vi "dust type.vi"(0 "Enable":bool=TRUE, 1 "Small?":bool, 2 "Sub vi?":bool, 5 "error in (no error)":errorcluster) -> (14 "Cancel 2":bool caption="Cancel", 15 "output cluster 2":T2 {"Batch" step=1; "Type" step=1; "Dust Source Builder:" items=["Keith Drake", "Nick Beaty", "Anthony Shu", "David James", "John Fontanese"]}, 16 "Dust Properties 2":T1, 18 "OK":bool, 19 "error out":errorcluster)   [LabVIEW 2013]
doc: "Displays a standard dialog box that prompts users to enter information, such as a user name and password.\n--------------------\n\nThis Express VI is configured as follows:\n\nMessage to Display to the User:Please Enter Experiment Settings Information For Database Storage.\nThe inputs are: \nNumber: Please Enter Group ID\nText Entry Box: Please Enter Tags:\nText Entry Box: Please Enter Experiment Description:"
uses:
  Controls/dust type.ctl
  Controls/source_builders.ctl
  Controls/dust_type_indicator.ctl
  <vilib>/Utility/miscctls.llb/LVPointTypeDef.ctl
  <vilib>/addons/database/Connection.llb/Conn Execute.vi
  <vilib>/addons/database/Recordset.llb/Rec Fetch Recordset Data (R).vi
  <vilib>/addons/database/Recordset.llb/Rec Destroy - Connection.vi
  <userlib>/_OpenG.lib/array/array.llb/Remove Duplicates from 1D Array (String)__ogtk.vi
  <userlib>/_OpenG.lib/array/array.llb/Search 1D Array (String)__ogtk.vi
  <userlib>/_OpenG.lib/array/array.llb/Index 1D Array Elements (I32)__ogtk.vi
  <userlib>/_OpenG.lib/array/array.llb/Conditional Auto-Indexing Tunnel (I32)__ogtk.vi
  <vilib>/addons/database/_DB Variant To Data/Database Variant To Data.xnode
  <vilib>/addons/database/NI_Database_API.lvlib
panel:
  in  "Transfer":bool caption="OK2"
  out "Comments":string[](array[string])
  out "Dust Properties":T1
  out "Dust Names":string[](array[string])
  out "Dust Weights":dbl[](array[numeric])
  out "Sizes":string[](array[string])
  out "Typical Weights":dbl[](array[numeric])
  out "Densities":dbl[](array[numeric])
  out "Batch Nos":i32[](array[numeric])
  out "Dust Types":i32[](array[numeric])
  out "Dust Type Ids":i32[](array[numeric])
  in  "Controls":T2 {"Batch" min=1 max=2 step=1; "Type" min=1 max=10 step=1; "Dust Source Builder:" items=["Keith Drake", "Nick Beaty", "Anthony Shu", "David James", "John Fontanese"]}
  in  "Create New":bool caption="OK2"
  in  "Cancel":bool
  in  "Update":bool caption="OK1"
  # "Please Enter Dust Information For Storage in the CCLDAS Database."
  # "Dust Information"
  # "Dust Information"
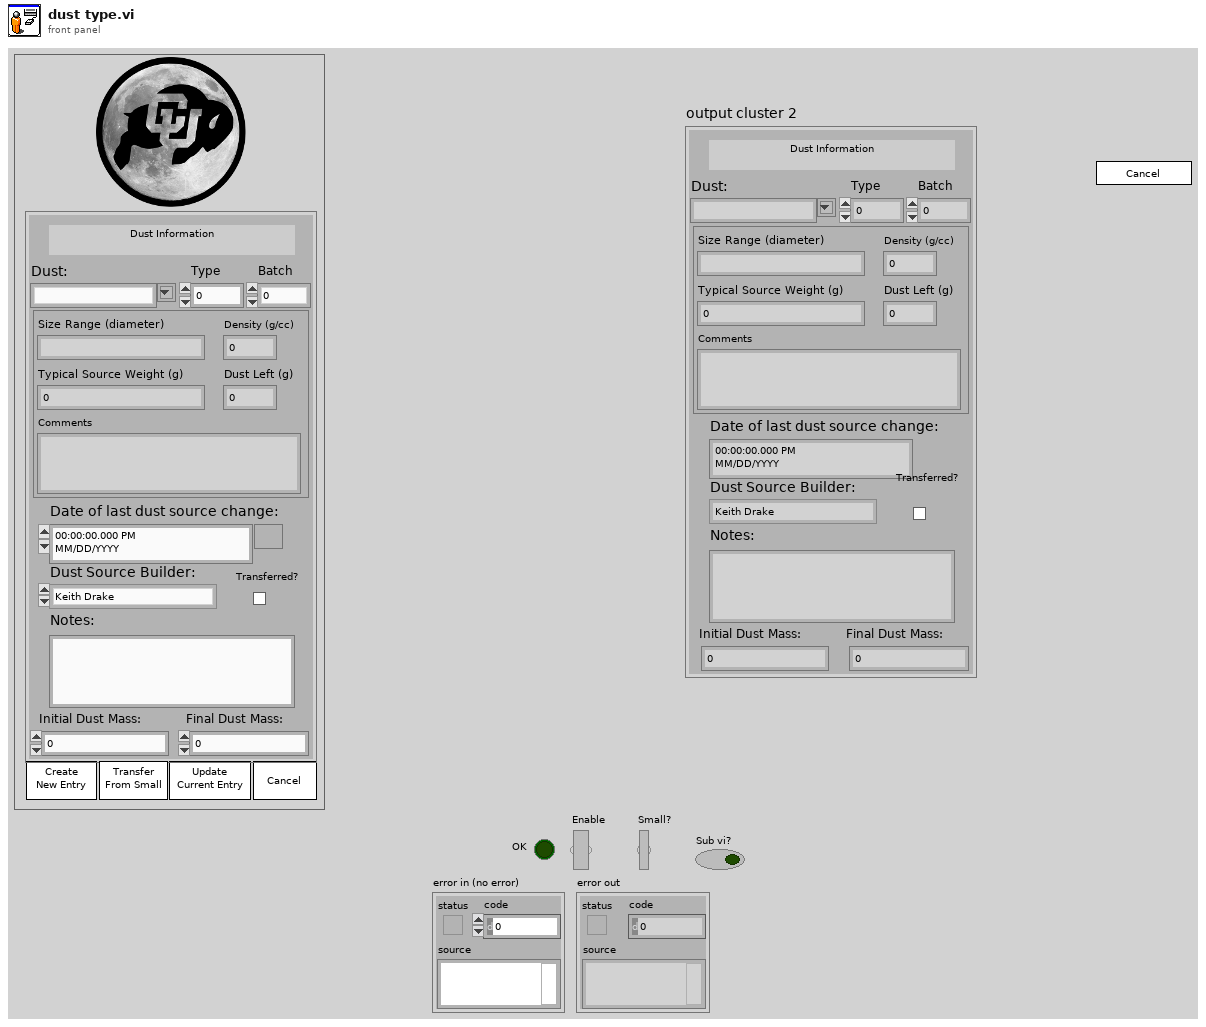
[diagram p1: front panel]
types:
  T1 = typedef "dust_type_indicator.ctl" = cluster{"Size Range (diameter)":string, "Density (g/cc)":dbl, "Typical Source Weight (g)":dbl, "Dust Left (g)":dbl, "Comments":string}
  T2 = typedef "dust type.ctl" = cluster{"Dust info id":u16, "Integer Timestamp":i64, "Dust:":string, "Dust Source Builder:":T3, "Notes:":string, "Date of last dust source change:":timestamp, "Initial Dust Mass:":dbl, "Final Dust Mass:":dbl, "Type":u16, "Batch":u16, "dust type id":u16, "Transferred?":bool}
  T3 = typedef "source_builders.ctl" = u16
  T4 = typedef "LVPointTypeDef.ctl" = cluster{"Horizontal":i16, "Vertical":i16}
  T5 = enum8{"Enabled", "Disabled", "Disabled and Grayed Out"}
  T6 = enum32{"Invalid", "Standard", "Closed", "Hidden", "Minimized", "Maximized"}
  T7 = cluster{"Dust info id":u16, "Integer Timestamp":i64, "dust type id":u16, "Dust Source Builder:":u16, "Notes:":string, "Initial Dust Mass:":dbl, "Final Dust Mass:":dbl, "shot count":u16, "run time":dbl, "From Small\nAccelerator":bool}
  T8 = typedef "NI_Database_API.lvlib/Conn ObjectReference.ctl" = refnum<k1>
  T9 = typedef "NI_Database_API.lvlib/Rec ObjectReference.ctl" = refnum<k1>
  T10 = cluster{"Dust event id":dbl, "Integer Time":i64, "dust type id":u16, "Dust Source Builder:":T3, "Notes:":string, "Initial Dust Mass:":dbl, "Dust event id":dbl, i16}
  T11 = cluster{"Dust event id":dbl, "Integer Time":i64, "dust type id":u16, "Dust Source Builder:":u16, "Notes:":string, "Initial Dust Mass:":dbl, "Final Dust Mass:":dbl, "shot count":u16, "run time":dbl, i16}
  T12 = cluster{"data":string, "data":dbl, "data":dbl, "data":dbl, "data":string}
  T13 = cluster{"Dust info id":u16, "Integer Timestamp":i64, "dust type id":u16, "Dust Source Builder:":T3, "Notes:":string, "Initial Dust Mass:":dbl, "Final Dust Mass:":dbl, i16}
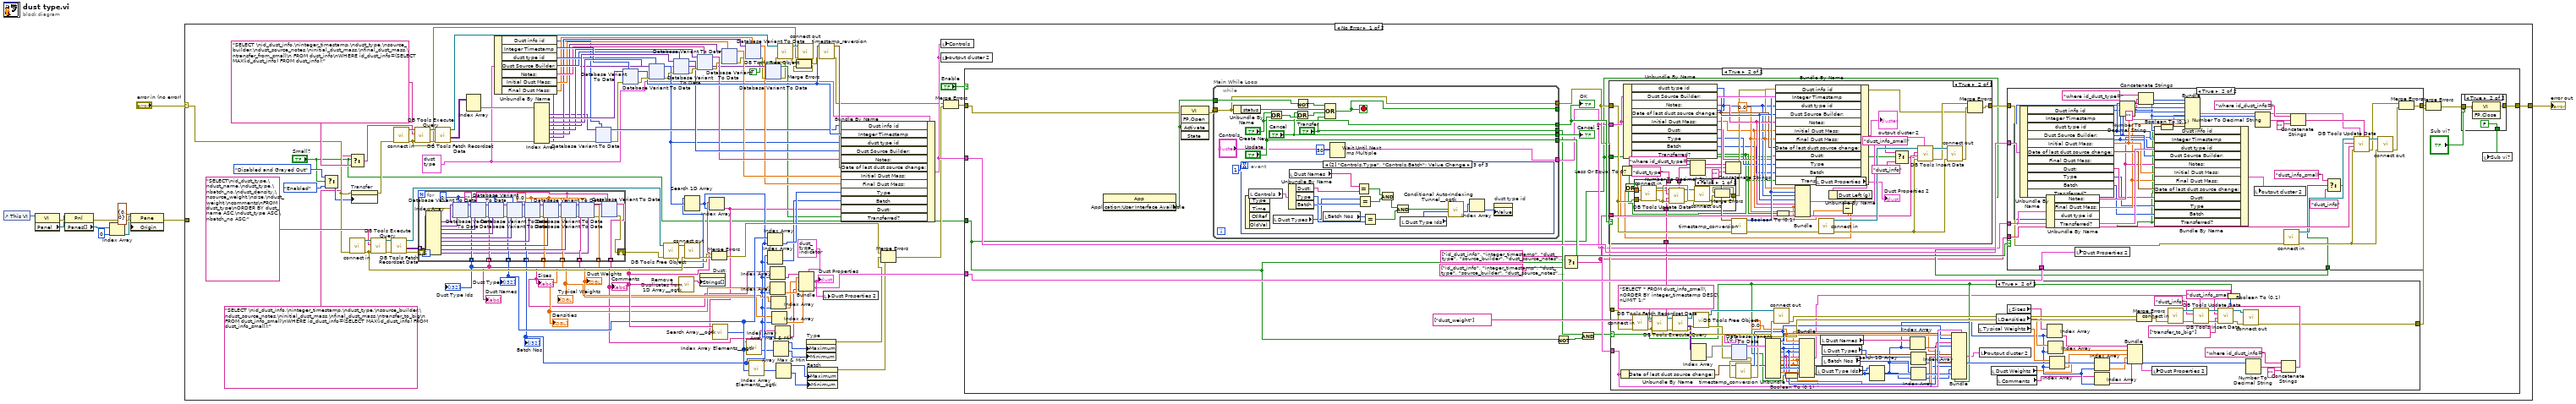
[diagram p0: block diagram]
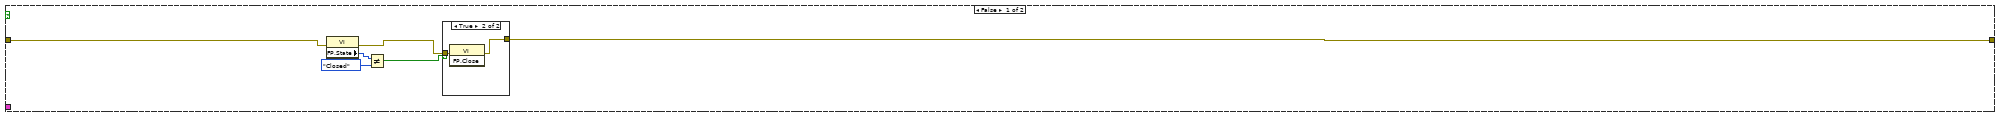
[diagram p2: hidden frame]
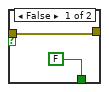
[diagram p4: hidden frame]
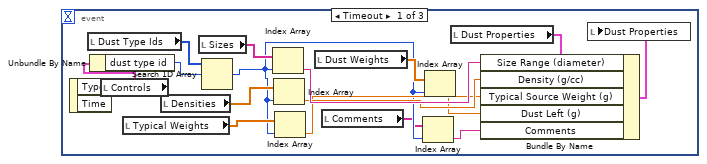
[diagram p7: hidden frame]
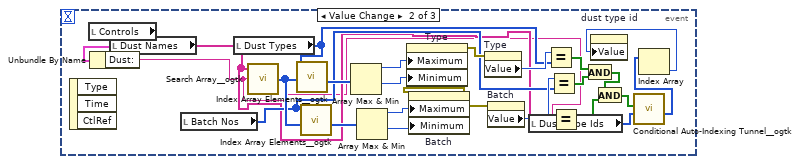
[diagram p8: hidden frame]
diagram:
  n1 = control-ref of="This VI"() -> (w9:refnum<vi>)
  n2 = property class="VI"(reference=w9) -> (error out=w8:errorcluster, "Panel"=w7:refnum<vi>)  [unwired: 1 in, 1 out]
  n3 = property class="Pnl"(reference=w7, error in=w8) -> (error out=w6:errorcluster, "Panes[]"=w5:refnum<vi>[])  [unwired: 1 out]
  n4 = Index Array(array=w5, index=0) -> (element=w3:refnum<vi>)
  n5 = property class="Pane"(reference=w3, error in=w6, "Origin"=T4 {"Horizontal"=0, "Vertical"=0}) -> (error out=w1:errorcluster)  [unwired: 1 out]
  n6 = case shown="No Error" "error in (no error)" {
    selector: "error in (no error)" -> [w25 w1275]
    tunnel: [w110 w1275] -> w10
    tunnel: w1 -> [_ _]
    frame No Error {
      w32 = T2 {"Dust info id"=0, "Integer Timestamp"=0, "Dust:"="", "Dust Source Builder:"=0, "Notes:"="", "Date of last dust source change:"=timestamp(0 s since 1904-01-01), "Initial Dust Mass:"=0.0, "Final Dust Mass:"=0.0, "Type"=0, "Batch"=0, "dust type id"=0, "Transferred?"=FALSE} ("Controls")
      n7 = Select(t=T5."Disabled and Grayed Out" ("Disabled"), s="Small?", f=T5."Enabled" ("Disabled")) -> (s? t:f=w21:T5)
      n8 = Select(t="SELECT \nid_dust_info,\ninteger_timestamp,\ndust_type,\nsource_builder,\ndust_source_notes,\ninitial_dust_mass,\nfinal_dust_mass,\ntransfer_to_big\n FROM dust_info_small\nWHERE id_dust_info=(SELECT MAX(id_dust_info) FROM dust_info_small);" ("SQL query"), s="Small?", f="SELECT \nid_dust_info,\ninteger_timestamp,\ndust_type,\nsource_builder,\ndust_source_notes,\ninitial_dust_mass,\nfinal_dust_mass,\ntransfer_from_small\n FROM dust_info\nWHERE id_dust_info=(SELECT MAX(id_dust_info) FROM dust_info);" ("SQL query")) -> (s? t:f=w26:string)
      n9 = call "connect in.vi"("error in (no error)"=w25) -> ("error out"=w69:errorcluster, "Database Connection"=w76:T8)  [unwired: 6 in, 1 out]
      n10 = property on="Transfer" class="Bool (strict)"(error in=w25, "DisabledEnum"=w21) -> (error out=w24:errorcluster)  [unwired: 1 in, 1 out]
      n11 = call-poly <vilib>:"DB Tools Execute Query.vi"("error in (no error)"=w69, "SQL query"="SELECT\nid_dust_type,\ndust_name,\ndust_type,\nbatch_no,\ndust_density,\nsource_weight,\nsize,\ndust_weight,\ncomments\nFROM dust_type\nORDER BY dust_name ASC,\ndust_type ASC,\nbatch_no ASC;", "connection reference"=w76) -> ("error out"=w78:errorcluster, "recordset reference"=w77:T9)  [unwired: 5 in]
      n12 = call-poly <vilib>:"DB Tools Fetch Recordset Data.vi"("error in (no error)"=w78, "recordset reference"=w77) -> ("error out"=w73:errorcluster, "recordset data"=w74:variant[][], "recordset reference out"=w70:T9)  [unwired: 3 in]
      n13 = call "connect in.vi"("error in (no error)"=w24) -> ("error out"=w68:errorcluster, "Database Connection"=w111:T8)  [unwired: 6 in, 1 out]
      n14 = call-poly <vilib>:"DB Tools Execute Query.vi"("error in (no error)"=w68, "SQL query"=w26, "connection reference"=w111) -> ("error out"=w113:errorcluster, "recordset reference"=w112:T9)  [unwired: 5 in]
      n15 = for {
        tunnel: w74 -> [w179] mode=indexing
        shift-right: [w149] -> w71
        shift-left: w73 -> [w170]
        tunnel: [w160] -> w61 mode=indexing
        tunnel: [w159] -> w59 mode=indexing
        tunnel: [w158] -> w57 mode=indexing
        tunnel: [w157] -> w56 mode=indexing
        tunnel: [w156] -> w53 mode=indexing
        tunnel: [w155] -> w54 mode=indexing
        tunnel: [w154] -> w52 mode=indexing
        tunnel: [w153] -> w55 mode=indexing
        tunnel: [w148] -> w34 mode=indexing
        w161 = 0.0
        w152 = ""
        w162 = 0
        n16 = Index Array(array=w179) -> (element #1=w178:variant, element #2=w177:variant, element #3=w176:variant, element #4=w175:variant, element #5=w174:variant, element #6=w173:variant, element #7=w172:variant, element #8=w171:variant, element #9=w151:variant)  [unwired: 9 in]
        n17 = xnode "Database Variant To Data"("database variant"=w178, "error in (no error)"=w170, "type"=w162) -> ("data"=w160:i32, "error out"=w169:errorcluster)
        n18 = xnode "Database Variant To Data"("database variant"=w177, "error in (no error)"=w169, "type"=w152) -> ("data"=w159:string, "error out"=w168:errorcluster)
        n19 = xnode "Database Variant To Data"("database variant"=w176, "error in (no error)"=w168, "type"=w162) -> ("data"=w158:i32, "error out"=w167:errorcluster)
        n20 = xnode "Database Variant To Data"("database variant"=w175, "error in (no error)"=w167, "type"=w162) -> ("data"=w157:i32, "error out"=w166:errorcluster)
        n21 = xnode "Database Variant To Data"("database variant"=w174, "error in (no error)"=w166, "type"=w161) -> ("data"=w156:dbl, "error out"=w165:errorcluster)
        n22 = xnode "Database Variant To Data"("database variant"=w173, "error in (no error)"=w165, "type"=w161) -> ("data"=w155:dbl, "error out"=w164:errorcluster)
        n23 = xnode "Database Variant To Data"("database variant"=w172, "error in (no error)"=w164, "type"=w152) -> ("data"=w154:string, "error out"=w163:errorcluster)
        n24 = xnode "Database Variant To Data"("database variant"=w171, "error in (no error)"=w163, "type"=w161) -> ("data"=w153:dbl, "error out"=w150:errorcluster)
        n25 = xnode "Database Variant To Data"("database variant"=w151, "error in (no error)"=w150, "type"=w152) -> ("data"=w148:string, "error out"=w149:errorcluster)
      }
      "Dust Type Ids" <- w61
      "Dust Types" <- w57
      "Batch Nos" <- w56
      "Densities" <- w53
      "Typical Weights" <- w54
      "Sizes" <- w52
      "Dust Weights" <- w55
      "Dust Names" <- w59
      "Comments" <- w34
      n26 = call-poly <vilib>:"DB Tools Fetch Recordset Data.vi"("error in (no error)"=w113, "recordset reference"=w112) -> ("error out"=w80:errorcluster, "recordset data"=w98:variant[][], "recordset reference out"=w114:T9)  [unwired: 3 in]
      n27 = Index Array(array=w98) -> (element=w97:variant[])  [unwired: 2 in]
      n28 = Unbundle By Name(w32) -> ("Dust info id"=w17:u16, "Integer Timestamp"=w104:i64, "dust type id"=w103:u16, "Dust Source Builder:"=w102:T3, "Notes:"=w100:string, "Initial Dust Mass:"=w89:dbl, "Final Dust Mass:"=w87:dbl)
      n29 = Index Array(array=w97) -> (element #1=w82:variant, element #2=w109:variant, element #3=w108:variant, element #4=w106:variant, element #5=w101:variant, element #6=w90:variant, element #7=w85:variant, element #8=w19:variant)  [unwired: 8 in]
      n30 = xnode "Database Variant To Data"("database variant"=w82, "error in (no error)"=w80, "type"=w17) -> ("data"=w81:u16, "error out"=w79:errorcluster)
      n31 = xnode "Database Variant To Data"("database variant"=w109, "error in (no error)"=w79, "type"=w104) -> ("data"=w95:i64, "error out"=w107:errorcluster)
      n32 = xnode "Database Variant To Data"("database variant"=w108, "error in (no error)"=w107, "type"=w103) -> ("data"=w62:u16, "error out"=w105:errorcluster)
      n33 = call-poly <vilib>:"DB Tools Free Object.vi"("error in (no error)"=w71, "recordset reference"=w70) -> ("error out"=w63:errorcluster, "connection reference"=w72:T8)  [unwired: 8 in]
      n34 = xnode "Database Variant To Data"("database variant"=w106, "error in (no error)"=w105, "type"=w102) -> ("data"=w92:T3, "error out"=w99:errorcluster)
      n35 = call-poly <userlib>:"Remove Duplicates from 1D Array__ogtk.vi"("Input Array"=w59) -> ("Output Array"=w60:string[])  [unwired: 1 out]
      n36 = call "connect out.vi"("error in (no error)"=w69, "connection reference"=w72) -> ("error out"=w64:errorcluster)  [unwired: 9 in]
      n37 = Search 1D Array(1D array=w61, element=w62) -> (index of element=w35:i32)  [unwired: 1 in]
      n38 = xnode "Database Variant To Data"("database variant"=w101, "error in (no error)"=w99, "type"=w100) -> ("data"=w91:string, "error out"=w84:errorcluster)
      n39 = property on="Dust:" class="CmbBox"("Strings[]"=w60) -> ()  [unwired: 2 in, 2 out]
      n40 = Index Array(array=w59, index=w35) -> (element=w28:string)
      n41 = Merge Errors(w63, w64) -> (w41:errorcluster)
      n42 = call-poly <userlib>:"Search Array__ogtk.vi"("Array"=w59, "Element Data"=w28) -> ("Indices of Elements"=w58:i32[])  [unwired: 7 in]
      n43 = xnode "Database Variant To Data"("database variant"=w90, "error in (no error)"=w84, "type"=w89) -> ("data"=w88:dbl, "error out"=w83:errorcluster)
      n44 = xnode "Database Variant To Data"("database variant"=w85, "error in (no error)"=w83, "type"=w87) -> ("data"=w86:dbl, "error out"=w14:errorcluster)
      n45 = call-poly <userlib>:"Index Array Elements__ogtk.vi"("indices"=w58, "array"=w57) -> ("elements"=w47:i32[])  [unwired: 9 in]
      n46 = call-poly <userlib>:"Index Array Elements__ogtk.vi"("indices"=w58, "array"=w56) -> ("elements"=w46:i32[])  [unwired: 9 in]
      n47 = xnode "Database Variant To Data"("database variant"=w19, "error in (no error)"=w14, "type"=TRUE ("Small?")) -> ("data"=w15:bool, "error out"=w13:errorcluster)
      n48 = Index Array(array=w56, index=w35) -> (element=w36:i32)
      n49 = Index Array(array=w57, index=w35) -> (element=w37:i32)
      n50 = Index Array(array=w52, index=w35) -> (element=w51:string)
      n51 = Index Array(array=w53, index=w35) -> (element=w50:dbl)
      n52 = Index Array(array=w54, index=w35) -> (element=w49:dbl)
      n53 = Index Array(array=w55, index=w35) -> (element=w48:dbl)
      n54 = Array Max & Min(array=w47) -> (max value=w45:i32, min value=w44:i32)  [unwired: 2 out]
      n55 = Index Array(array=w34, index=w35) -> (element=w33:string)
      n56 = Array Max & Min(array=w46) -> (max value=w43:i32, min value=w42:i32)  [unwired: 2 out]
      n57 = call-poly <vilib>:"DB Tools Free Object.vi"("error in (no error)"=w13, "recordset reference"=w114) -> ("error out"=w67:errorcluster, "connection reference"=w115:T8)  [unwired: 8 in]
      n58 = call "connect out.vi"("error in (no error)"=w68, "connection reference"=w115) -> ("error out"=w65:errorcluster)  [unwired: 9 in]
      n59 = Merge Errors(w67, w65) -> (w66:errorcluster)
      n60 = Bundle(cluster=T1 {"Size Range (diameter)"="60 nm - 10 µm", "Density (g/cc)"=7874.0, "Typical Source Weight (g)"=1.2000000476837158, "Dust Left (g)"=0.9300000071525574, "Comments"="8:1 mix of Iron-8-1 and Iron-4-1."} ("Dust Properties"), "Size Range (diameter)"=w51, "Density (g/cc)"=w50, "Typical Source Weight (g)"=w49, "Dust Left (g)"=w48, "Comments"=w33) -> (w31:T1)
      "Dust Properties" <- w31
      n61 = property on="Type" class="DigNum (strict)"("Maximum"=w45, "Minimum"=w44) -> (error out=w30:errorcluster)  [unwired: 2 in, 1 out]
      n62 = property on="Batch" class="DigNum (strict)"("Maximum"=w43, "Minimum"=w42) -> (error out=w29:errorcluster)  [unwired: 2 in, 1 out]
      n63 = call "timestamp_reversion.vi"("error in (no error)"=w66, "Integer Timestamp"=w95) -> ("error out"=w39:errorcluster, "time stamp"=w93:timestamp)  [unwired: 7 in]
      n64 = local write "Dust Properties 2"(w31) -> ()
      n65 = Bundle By Name(cluster=w32, "Dust info id"=w81, "Integer Timestamp"=w95, "dust type id"=w62, "Dust Source Builder:"=w92, "Notes:"=w91, "Date of last dust source change:"=w93, "Initial Dust Mass:"=w88, "Final Dust Mass:"=w86, "Type"=w37, "Batch"=w36, "Dust:"=w28, "Transferred?"=w15) -> (w94:T2)
      n66 = Merge Errors(w41, w30, w29) -> (w38:errorcluster)
      n67 = local write "Controls"(w94) -> ()
      n68 = local write "output cluster 2"(w94) -> ()
      n69 = Merge Errors(w39, w38) -> (w40:errorcluster)
      n70 = case shown="True" "Enable" {
        tunnel: w40 -> [w568 w582]
        tunnel: [w569 w596] -> w110
        tunnel: w94 -> [_ w592]
        tunnel: w31 -> [_ w589]
        tunnel: "Small?" -> [_ w578]
        frame False {
          n71 = property class="VI"(error in=w568) -> (error out=w567:errorcluster, "FP.State"=w566:T6)  [unwired: 1 in, 1 out]
          n72 = Not Equal?(x=w566, y=T6."Closed") -> (x != y?=w564:bool)
          n73 = case shown="True" w564 {
            tunnel: [w570 w572] -> w569
            tunnel: w567 -> [w570 w571]
            frame False {
            }
            frame True {
              n74 = invoke class="VI" method="FP.Close"(error in=w571) -> (error out=w572:errorcluster)  [unwired: 2 in, 2 out]
            }
          }
        }
        frame True {
          n75 = property class="App"() -> ("Application:User Interface Available"=w591:bool)  [unwired: 2 in, 2 out]
          n76 = invoke class="VI" method="FP.Open"(error in=w582, "Activate"=w591) -> (error out=w597:errorcluster)  [unwired: 3 in, 4 out]
          n77 = while "Main While Loop" {
            tunnel: w591 -> [w1036]
            tunnel: [w1032] -> _
            tunnel: w597 -> [w1030]
            tunnel: [w1030] -> w587
            tunnel: ["Cancel"] -> w595
            tunnel: ["Controls"] -> w586
            tunnel: ["Update"] -> w594
            tunnel: ["Create New"] -> w588
            tunnel: ["Transfer"] -> w579
            stop <- w1032 stop-if-true
            n78 = Unbundle By Name(w1030) -> ("status"=w1033:bool)
            n79 = event shown="[2] \"Controls.Type\", \"Controls.Batch\": Value Change" {
              selector: _ -> [_ _ _]
              dyn-events: _ -> [_ _ _]
              timeout: 1 -> [_ _ _]
              event Timeout {
                n80 = event-data() -> ()  [unwired: 1 in, 2 out]
                n81 = local read "Dust Type Ids"() -> (w1053:i32[])
                n82 = local read "Controls"() -> (w1039:T2)
                n83 = Unbundle By Name(w1039) -> ("dust type id"=w1054:u16)
                n84 = local read "Typical Weights"() -> (w1050:dbl[])
                n85 = local read "Densities"() -> (w1051:dbl[])
                n86 = local read "Sizes"() -> (w1052:string[])
                n87 = Search 1D Array(1D array=w1053, element=w1054) -> (index of element=w1042:i32)  [unwired: 1 in]
                n88 = Index Array(array=w1052, index=w1042) -> (element=w1046:string)
                n89 = Index Array(array=w1051, index=w1042) -> (element=w1045:dbl)
                n90 = Index Array(array=w1050, index=w1042) -> (element=w1044:dbl)
                n91 = local read "Dust Weights"() -> (w1049:dbl[])
                n92 = local read "Comments"() -> (w1041:string[])
                n93 = Index Array(array=w1041, index=w1042) -> (element=w1040:string)
                n94 = Index Array(array=w1049, index=w1042) -> (element=w1043:dbl)
                n95 = local read "Dust Properties"() -> (w1047:T1)
                n96 = Bundle By Name(cluster=w1047, "Size Range (diameter)"=w1046, "Density (g/cc)"=w1045, "Typical Source Weight (g)"=w1044, "Dust Left (g)"=w1043, "Comments"=w1040) -> (w1048:T1)
                n97 = local write "Dust Properties"(w1048) -> ()
              }
              event Value Change {
                n98 = event-data() -> ()  [unwired: 1 in, 3 out]
                n99 = local read "Controls"() -> (w1056:T2)
                n100 = Unbundle By Name(w1056) -> ("Dust:"=w1055:string)
                n101 = local read "Dust Names"() -> (w1065:string[])
                n102 = local read "Batch Nos"() -> (w1066:i32[])
                n103 = local read "Dust Types"() -> (w1068:i32[])
                n104 = call-poly <userlib>:"Search Array__ogtk.vi"("Array"=w1065, "Element Data"=w1055) -> ("Indices of Elements"=w1077:i32[])  [unwired: 7 in]
                n105 = call-poly <userlib>:"Index Array Elements__ogtk.vi"("indices"=w1077, "array"=w1068) -> ("elements"=w1076:i32[])  [unwired: 9 in]
                n106 = call-poly <userlib>:"Index Array Elements__ogtk.vi"("indices"=w1077, "array"=w1066) -> ("elements"=w1078:i32[])  [unwired: 9 in]
                n107 = Array Max & Min(array=w1076) -> (max value=w1075:i32, min value=w1074:i32)  [unwired: 2 out]
                n108 = Array Max & Min(array=w1078) -> (max value=w1073:i32, min value=w1072:i32)  [unwired: 2 out]
                n109 = property on="Type" class="DigNum (strict)"("Maximum"=w1075, "Minimum"=w1074) -> (error out=w1071:errorcluster)  [unwired: 2 in, 1 out]
                n110 = property on="Batch" class="DigNum (strict)"("Maximum"=w1073, "Minimum"=w1072) -> (error out=w1070:errorcluster)  [unwired: 2 in, 1 out]
                n111 = property on="Type" class="DigNum (strict)"(error in=w1071) -> ("Value"=w1069:u16)  [unwired: 1 in, 2 out]
                n112 = property on="Batch" class="DigNum (strict)"(error in=w1070) -> ("Value"=w1067:u16)  [unwired: 1 in, 2 out]
                n113 = local read "Dust Type Ids"() -> (w1059:i32[])
                n114 = Equal?(x=w1069, y=w1068) -> (x = y?=w1064:bool[])
                n115 = Equal?(x=w1067, y=w1066) -> (x = y?=w1063:bool[])
                n116 = Equal?(x=w1055, y=w1065) -> (x = y?=w1061:bool[])
                n117 = And(x=w1064, y=w1063) -> (x .and. y?=w1062:bool[])
                n118 = And(x=w1062, y=w1061) -> (x .and. y?=w1060:bool[])
                n119 = call-poly <userlib>:"Conditional Auto-Indexing Tunnel__ogtk.vi"("Array in"=w1059, "Elements to keep"=w1060) -> ("Filtered Array out"=w1058:i32[])  [unwired: 5 in]
                n120 = Index Array(array=w1058) -> (element=w1057:i32)  [unwired: 1 in]
                n121 = property on="dust type id" class="Ring (strict)"("Value"=w1057) -> ()  [unwired: 2 in, 2 out]
              }
              event Value Change {
                n122 = event-data() -> ()  [unwired: 1 in, 4 out]
                n123 = local read "Controls"() -> (w1080:T2)
                n124 = local read "Dust Types"() -> (w1089:i32[])
                n125 = Unbundle By Name(w1080) -> ("Dust:"=w1079:string, "Type"=w1093:u16, "Batch"=w1092:u16)
                n126 = local read "Dust Names"() -> (w1091:string[])
                n127 = local read "Batch Nos"() -> (w1090:i32[])
                n128 = Equal?(x=w1091, y=w1079) -> (x = y?=w1088:bool[])
                n129 = Equal?(x=w1089, y=w1093) -> (x = y?=w1087:bool[])
                n130 = Equal?(x=w1090, y=w1092) -> (x = y?=w1085:bool[])
                n131 = And(x=w1088, y=w1087) -> (x .and. y?=w1086:bool[])
                n132 = And(x=w1086, y=w1085) -> (x .and. y?=w1084:bool[])
                n133 = local read "Dust Type Ids"() -> (w1083:i32[])
                n134 = call-poly <userlib>:"Conditional Auto-Indexing Tunnel__ogtk.vi"("Array in"=w1083, "Elements to keep"=w1084) -> ("Filtered Array out"=w1082:i32[])  [unwired: 5 in]
                n135 = Index Array(array=w1082) -> (element=w1081:i32)  [unwired: 1 in]
                n136 = property on="dust type id" class="Ring (strict)"("Value"=w1081) -> ()  [unwired: 2 in, 2 out]
              }
            }
            n137 = Or(x="Create New", y="Update") -> (x .or. y?=w1037:bool)
            n138 = Or(x="Cancel", y=w1037) -> (x .or. y?=w1034:bool)
            n139 = Not(x=w1036) -> (.not. x?=w1035:bool)
            n140 = Compound Arithmetic op=OR(w1035, w1033, w1034, "Transfer") -> (w1032:bool)
            n141 = Wait Until Next ms Multiple(millisecond multiple=u32 50) -> ()  [unwired: 1 out]
          }
          "OK" <- w588
          "Cancel 2" <- w595
          n142 = Not(x=w578) -> (.not. x?=w580:bool)
          n143 = Select(t=string[] ["id_dust_info", "integer_timestamp", "dust_type", "source_builder", "dust_source_notes", "initial_dust_mass", "final_dust_mass", "transfer_to_big"] ("columns"), s=w578, f=string[] ["id_dust_info", "integer_timestamp", "dust_type", "source_builder", "dust_source_notes", "initial_dust_mass", "final_dust_mass", "transfer_from_small"] ("columns")) -> (s? t:f=w575:string[])
          n144 = And(x=w579, y=w580) -> (x .and. y?=w581:bool)
          n145 = case shown="True" w588 {
            tunnel: w587 -> [w1094 w1118]
            tunnel: [w1094 w1122] -> w593
            tunnel: w586 -> [_ w1128]
            tunnel: w575 -> [_ w1121]
            tunnel: string[] ["dust_weight"] -> [_ w1116]
            tunnel: w578 -> [_ w1097]
            frame False {
            }
            frame True {
              w1119 = 0.0 ("Dust event id")
              n146 = Unbundle By Name(w1128) -> ("dust type id"=w1105:u16, "Dust Source Builder:"=w1125:T3, "Notes:"=w1124:string, "Date of last dust source change:"=w1120:timestamp, "Initial Dust Mass:"=w1113:dbl, "Dust:"=w1104:string, "Type"=w1103:u16, "Batch"=w1102:u16, "Transferred?"=w1100:bool)
              n147 = Number To Decimal String(number=w1105) -> (decimal integer string=w1108:string)  [unwired: 1 in]
              n148 = Concatenate Strings("where id_dust_type=" ("condition"), w1108, "" ("string")) -> (w1106:string)
              n149 = call "timestamp_conversion.vi"("error in (no error)"=w1118, "Time Stamp"=w1120) -> ("error out"=w1134:errorcluster, "Integer Time"=w1126:i64)  [unwired: 7 in]
              n150 = Bundle By Name(cluster=w1128, "Dust info id"=w1119, "Integer Timestamp"=w1126, "dust type id"=w1105, "Dust Source Builder:"=w1125, "Notes:"=w1124, "Initial Dust Mass:"=w1113, "Final Dust Mass:"=w1119, "Date of last dust source change:"=w1120, "Dust:"=w1104, "Type"=w1103, "Batch"=w1102, "Transferred?"=w1100) -> (→"output cluster 2":T2)
              n151 = Boolean To (0,1)(Boolean=w1100) -> (0, 1=w1095:i16)
              n152 = Bundle("Dust event id"=w1119, "Integer Time"=w1126, "dust type id"=w1105, "Dust Source Builder:"=w1125, "Notes:"=w1124, "Initial Dust Mass:"=w1113, "Dust event id"=w1119, w1095) -> (w1123:T10)  [unwired: 1 in]
              n153 = local read "Dust Properties"() -> (w1114:T1)
              "Dust Properties 2" <- w1114
              n154 = call "connect in.vi"("error in (no error)"=w1134) -> ("error out"=w1131:errorcluster, "Database Connection"=w1133:T8)  [unwired: 6 in, 1 out]
              n155 = Unbundle By Name(w1114) -> ("Dust Left (g)"=w1110:dbl)
              n156 = Less Or Equal To 0?(x=w1110) -> (x <= 0?=w1111:bool)
              n157 = Or(x=w1111, y=w1100) -> (x .or. y?=w1101:bool)
              n158 = Subtract(x=w1110, y=w1113) -> (x-y=w1112:dbl)
              n159 = case shown="False" w1101 {
                tunnel: [w1142 w1146] -> w1117
                tunnel: w1118 -> [w1141 w1146]
                tunnel: w1116 -> [w1140 _]
                tunnel: "dust_type" -> [w1139 _]
                tunnel: w1112 -> [w1136 _]
                tunnel: w1106 -> [w1135 _]
                frame False {
                  n160 = call "connect in.vi"("error in (no error)"=w1141) -> ("error out"=w1145:errorcluster, "Database Connection"=w1138:T8)  [unwired: 6 in, 1 out]
                  n161 = call <vilib>:"DB Tools Update Data.vi"("condition"=w1135, "data"=w1136, "error in (no error)"=w1145, "columns"=w1140, "table"=w1139, "connection reference"=w1138) -> ("error out"=w1144:errorcluster, "connection reference out"=w1137:T8)  [unwired: 4 in]
                  n162 = call "connect out.vi"("error in (no error)"=w1145, "connection reference"=w1137) -> ("error out"=w1143:errorcluster)  [unwired: 9 in]
                  n163 = Merge Errors(w1143, w1144) -> (w1142:errorcluster)
                }
                frame True {
                }
              }
              n164 = Select(t="dust_info_small" ("table"), s=w1097, f="dust_info" ("table")) -> (s? t:f=w1096:string)
              n165 = call <vilib>:"DB Tools Insert Data.vi"("data"=w1123, "error in (no error)"=w1131, "columns"=w1121, "table"=w1096, "connection reference"=w1133) -> ("error out"=w1130:errorcluster, "connection reference out"=w1132:T8)  [unwired: 5 in]
              n166 = call "connect out.vi"("error in (no error)"=w1131, "connection reference"=w1132) -> ("error out"=w1129:errorcluster)  [unwired: 9 in]
              n167 = Merge Errors(w1130, w1129, w1117) -> (w1122:errorcluster)
            }
          }
          n168 = case shown="True" w581 {
            selector: w581 -> [_ w620]
            tunnel: w587 -> [w603 w669]
            tunnel: w586 -> [_ w636]
            tunnel: [w603 w637] -> w583
            frame False {
            }
            frame True {
              w635 = 0.0 ("Dust event id")
              n169 = Unbundle By Name(w636) -> ("Date of last dust source change:"=w625:timestamp)
              n170 = call "connect in.vi"("error in (no error)"=w669) -> ("error out"=w667:errorcluster, "Database Connection"=w668:T8)  [unwired: 6 in, 1 out]
              n171 = call-poly <vilib>:"DB Tools Execute Query.vi"("error in (no error)"=w667, "SQL query"="SELECT * FROM dust_info_small\nORDER BY integer_timestamp DESC\nLIMIT 1;", "connection reference"=w668) -> ("error out"=w671:errorcluster, "recordset reference"=w670:T9)  [unwired: 5 in]
              n172 = call-poly <vilib>:"DB Tools Fetch Recordset Data.vi"("error in (no error)"=w671, "recordset reference"=w670) -> ("error out"=w665:errorcluster, "recordset data"=w662:variant[][], "recordset reference out"=w666:T9)  [unwired: 3 in]
              n173 = Index Array(array=w662) -> (element=w661:variant[])  [unwired: 2 in]
              n174 = call-poly <vilib>:"DB Tools Free Object.vi"("error in (no error)"=w665, "recordset reference"=w666) -> ("error out"=w660:errorcluster, "connection reference"=w664:T8)  [unwired: 8 in]
              n175 = xnode "Database Variant To Data"("database variant"=w661, "error in (no error)"=w660, "type"=T7 {"Dust info id"=0, "Integer Timestamp"=0, "dust type id"=0, "Dust Source Builder:"=0, "Notes:"="", "Initial Dust Mass:"=0.0, "Final Dust Mass:"=0.0, "shot count"=0, "run time"=0.0, "From Small\nAccelerator"=FALSE}) -> ("data"=w656:T7, "error out"=w652:errorcluster)
              n176 = call "timestamp_conversion.vi"("error in (no error)"=w652, "Time Stamp"=w625) -> ("error out"=w639:errorcluster, "Integer Time"=w634:i64)  [unwired: 7 in]
              n177 = Unbundle(w656) -> ("Dust info id"=w644:u16, "dust type id"=w633:u16, "Dust Source Builder:"=w627:u16, "Notes:"=w626:string, "Initial Dust Mass:"=w624:dbl, "Final Dust Mass:"=w623:dbl, "shot count"=w654:u16, "run time"=w653:dbl)  [unwired: 2 out]
              n178 = call "connect out.vi"("error in (no error)"=w667, "connection reference"=w664) -> ("error out"=w640:errorcluster)  [unwired: 9 in]
              n179 = Boolean To (0,1)(Boolean=w620) -> (0, 1=w605:i16)
              n180 = Bundle("Dust event id"=w635, "Integer Time"=w634, "dust type id"=w633, "Dust Source Builder:"=w627, "Notes:"=w626, "Initial Dust Mass:"=w624, "Final Dust Mass:"=w623, "shot count"=w654, "run time"=w653, w605) -> (w604:T11)  [unwired: 1 in]
              n181 = local read "Dust Type Ids"() -> (w632:i32[])
              n182 = local read "Dust Names"() -> (w631:string[])
              n183 = local read "Dust Types"() -> (w630:i32[])
              n184 = local read "Batch Nos"() -> (w629:i32[])
              n185 = Search 1D Array(1D array=w632, element=w633) -> (index of element=w612:i32)  [unwired: 1 in]
              n186 = Index Array(array=w631, index=w612) -> (element=w628:string)
              n187 = Index Array(array=w630, index=w612) -> (element=w622:i32)
              n188 = Index Array(array=w629, index=w612) -> (element=w621:i32)
              n189 = Bundle(cluster=w636, "Dust info id"=w635, "Integer Timestamp"=w634, "Dust:"=w628, "Dust Source Builder:"=w627, "Notes:"=w626, "Date of last dust source change:"=w625, "Initial Dust Mass:"=w624, "Final Dust Mass:"=w623, "Type"=w622, "Batch"=w621, "dust type id"=w633, "Transferred?"=w620) -> (w619:T2)
              n190 = local read "Typical Weights"() -> (w616:dbl[])
              n191 = local write "output cluster 2"(w619) -> ()
              n192 = local read "Dust Weights"() -> (w611:dbl[])
              n193 = local read "Densities"() -> (w617:dbl[])
              n194 = local read "Comments"() -> (w610:string[])
              n195 = local read "Sizes"() -> (w618:string[])
              n196 = Index Array(array=w618, index=w612) -> (element=w615:string)
              n197 = Index Array(array=w617, index=w612) -> (element=w614:dbl)
              n198 = Index Array(array=w616, index=w612) -> (element=w613:dbl)
              n199 = Index Array(array=w610, index=w612) -> (element=w608:string)
              n200 = Index Array(array=w611, index=w612) -> (element=w609:dbl)
              n201 = Bundle("data"=w615, "data"=w614, "data"=w613, "data"=w609, "data"=w608) -> (w607:T12)  [unwired: 1 in]
              n202 = Merge Errors(w640, w639) -> (w638:errorcluster)
              n203 = local write "Dust Properties 2"(w607) -> ()
              n204 = call "connect in.vi"("error in (no error)"=w638) -> ("error out"=w658:errorcluster, "Database Connection"=w659:T8)  [unwired: 6 in, 1 out]
              n205 = call <vilib>:"DB Tools Insert Data.vi"("data"=w604, "error in (no error)"=w658, "table"="dust_info", "connection reference"=w659) -> ("error out"=w649:errorcluster, "connection reference out"=w651:T8)  [unwired: 6 in]
              n206 = Boolean To (0,1)(Boolean=w620) -> (0, 1=w606:i16)
              n207 = Number To Decimal String(number=w644) -> (decimal integer string=w646:string)  [unwired: 1 in]
              n208 = Concatenate Strings("where id_dust_info=" ("condition"), w646, "" ("string")) -> (w643:string)
              n209 = call <vilib>:"DB Tools Update Data.vi"("condition"=w643, "data"=w606, "error in (no error)"=w649, "columns"=string[] ["transfer_to_big"], "table"="dust_info_small", "connection reference"=w651) -> ("error out"=w642:errorcluster, "connection reference out"=w641:T8)  [unwired: 4 in]
              n210 = call "connect out.vi"("error in (no error)"=w642, "connection reference"=w641) -> ("error out"=w637:errorcluster)  [unwired: 9 in]
            }
          }
          n211 = case shown="True" w594 {
            tunnel: [w986 w1018] -> w584
            tunnel: w593 -> [w986 w1002]
            tunnel: w575 -> [_ w1024]
            tunnel: w586 -> [_ w1011]
            tunnel: w592 -> [_ w1012]
            tunnel: w589 -> [_ w993]
            tunnel: w578 -> [_ w991]
            frame False {
            }
            frame True {
              n212 = Unbundle By Name(w1012) -> ("Dust info id"=w1006:u16, "Integer Timestamp"=w1007:i64, "dust type id"=w1008:u16, "Dust Source Builder:"=w1009:T3, "Initial Dust Mass:"=w1010:dbl, "Date of last dust source change:"=w1005:timestamp, "Dust:"=w996:string, "Type"=w995:u16, "Batch"=w994:u16)  [unwired: 2 out]
              n213 = Unbundle By Name(w1011) -> ("Notes:"=w1003:string, "Final Dust Mass:"=w1001:dbl, "dust type id"=w997:u16, "Transferred?"=w988:bool)
              n214 = local write "Dust Properties 2"(w993) -> ()
              n215 = Number To Decimal String(number=w997) -> (decimal integer string=w999:string)  [unwired: 1 in]
              n216 = Concatenate Strings("where id_dust_type=" ("condition"), w999, "" ("string")) -> ()  [unwired: 1 out]
              n217 = Bundle By Name(cluster=w1011, "Dust info id"=w1006, "Integer Timestamp"=w1007, "dust type id"=w1008, "Dust Source Builder:"=w1009, "Notes:"=w1003, "Initial Dust Mass:"=w1010, "Final Dust Mass:"=w1001, "Date of last dust source change:"=w1005, "Dust:"=w996, "Type"=w995, "Batch"=w994, "Transferred?"=w988) -> (w1013:T2)
              n218 = Boolean To (0,1)(Boolean=w988) -> (0, 1=w987:i16)
              n219 = Bundle("Dust info id"=w1006, "Integer Timestamp"=w1007, "dust type id"=w1008, "Dust Source Builder:"=w1009, "Notes:"=w1003, "Initial Dust Mass:"=w1010, "Final Dust Mass:"=w1001, w987) -> (w1004:T13)  [unwired: 1 in]
              n220 = local write "output cluster 2"(w1013) -> ()
              n221 = Number To Decimal String(number=w1006) -> (decimal integer string=w1016:string)  [unwired: 1 in]
              n222 = call "connect in.vi"("error in (no error)"=w1002) -> ("error out"=w1019:errorcluster, "Database Connection"=w1023:T8)  [unwired: 6 in, 1 out]
              n223 = Concatenate Strings("where id_dust_info=" ("condition"), w1016, "" ("string")) -> (w1014:string)
              n224 = Select(t="dust_info_small" ("table"), s=w991, f="dust_info" ("table")) -> (s? t:f=w990:string)
              n225 = call <vilib>:"DB Tools Update Data.vi"("condition"=w1014, "data"=w1004, "error in (no error)"=w1019, "columns"=w1024, "table"=w990, "connection reference"=w1023) -> ("error out"=w1021:errorcluster, "connection reference out"=w1022:T8)  [unwired: 4 in]
              n226 = call "connect out.vi"("error in (no error)"=w1019, "connection reference"=w1022) -> ("error out"=w1020:errorcluster)  [unwired: 9 in]
              n227 = Merge Errors(w1021, w1020) -> (w1018:errorcluster)
            }
          }
          n228 = Merge Errors(w584, w583) -> (w585:errorcluster)
          n229 = case shown="True" "Sub vi?" {
            tunnel: [w599 w602] -> w596
            tunnel: w585 -> [w599 w601]
            tunnel: [FALSE ("Sub vi?") FALSE ("Sub vi?")] -> w573
            frame False {
            }
            frame True {
              n230 = invoke class="VI" method="FP.Close"(error in=w601) -> (error out=w602:errorcluster)  [unwired: 2 in, 2 out]
            }
          }
          n231 = local write "Sub vi?"(w573) -> ()
        }
      }
    }
    frame Error {
    }
  }
  "error out" <- w10
